vi "内泄露.vi"(0 "内泄漏曲线":refnum<vi>, 1 "内泄漏":cluster{"下限":dbl, "上限":dbl}, 3 "错误输入":errorcluster) -> (8 "OK？":bool, 10 "错误输出":errorcluster)   [LabVIEW 2018]
uses:
  Global_Variable/Global.vi
  Global_Variable/A180648.vi
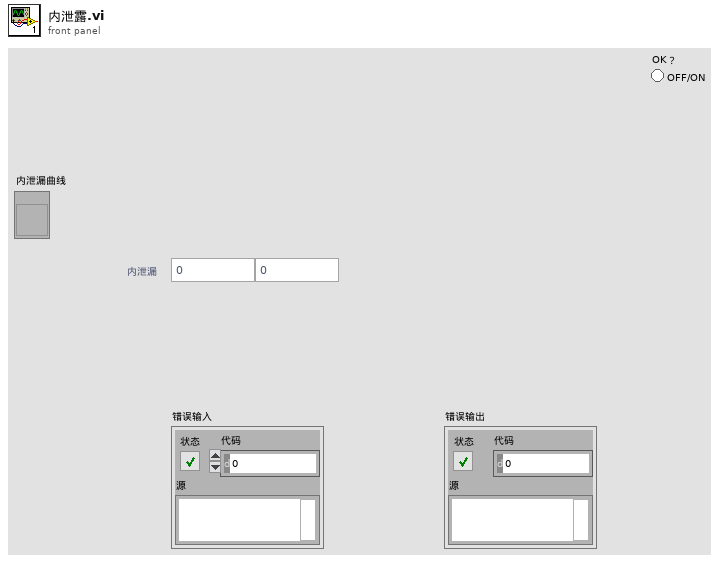
[diagram p1: front panel]
types:
  T1 = enum32{"空载", "功能", "力特性", "传感器特性", "电流特性", "振动NVH", "逆向空载", "完成"}
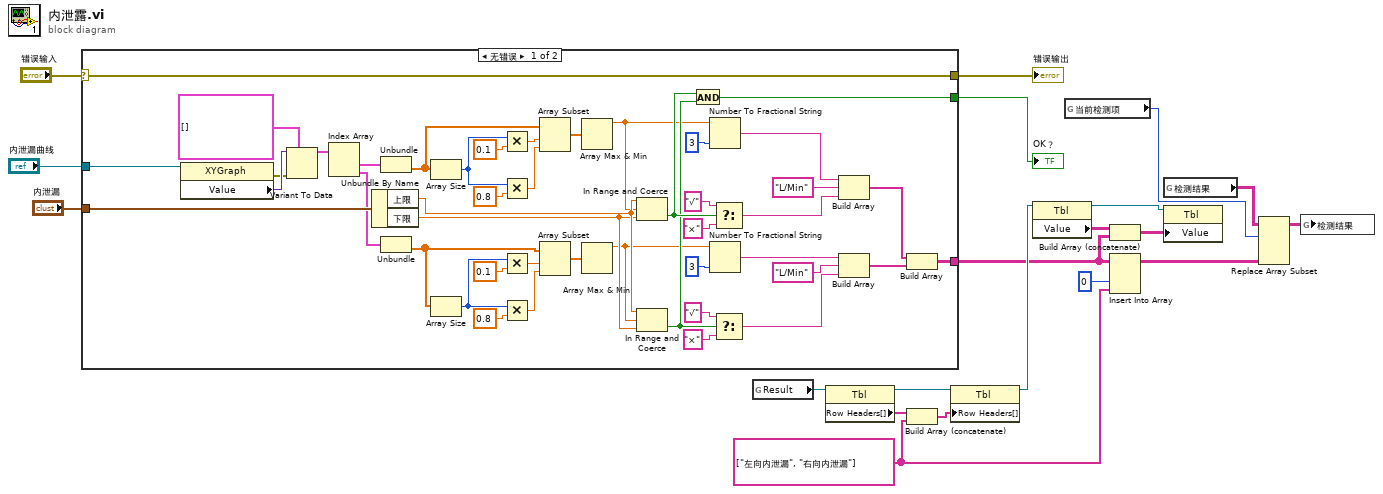
[diagram p0: block diagram]
diagram:
  w3 = string[] ["左向内泄漏", "右向内泄漏"] ("列首字符串[]")
  n1 = case shown="无错误" "错误输入" {
    selector: "错误输入" -> [w44 w66]
    tunnel: [w44 w66] -> w19
    tunnel: [w46 _] -> w18
    tunnel: "内泄漏" -> [w58 _]
    tunnel: [w59 _] -> w4
    tunnel: "内泄漏曲线" -> [w39 _]
    frame No Error {
      n2 = property class="XYGraph"(reference=w39) -> (error out=w42:errorcluster, "Value"=w43:variant)  [unwired: 1 in, 1 out]
      n3 = Variant To Data(error in=w42, type=cluster{dbl[], dbl[]}[] [], Variant=w43) -> (data=w41:cluster{dbl[], dbl[]}[])  [unwired: 1 out]
      n4 = Index Array(array=w41) -> (element #1=w38:cluster{dbl[], dbl[]}, element #2=w37:cluster{dbl[], dbl[]})  [unwired: 2 in]
      n5 = Unbundle By Name(w58) -> ("上限"=w51:dbl, "下限"=w50:dbl)
      n6 = Unbundle(w38) -> (w35:dbl[])  [unwired: 1 out]
      n7 = Unbundle(w37) -> (w23:dbl[])  [unwired: 1 out]
      n8 = Array Size(array=w35) -> (size(s)=w32:i32)
      n9 = Array Size(array=w23) -> (size(s)=w24:i32)
      n10 = Multiply(x=w32, y=0.1) -> (x*y=w30:dbl)
      n11 = Multiply(x=w32, y=0.8) -> (x*y=w29:dbl)
      n12 = Multiply(x=w24, y=0.1) -> (x*y=w26:dbl)
      n13 = Multiply(x=w24, y=0.8) -> (x*y=w27:dbl)
      n14 = Array Subset(array=w35, index=w30, length=w29) -> (w28:dbl[])
      n15 = Array Subset(array=w23, index=w26, length=w27) -> (w21:dbl[])
      n16 = Array Max & Min(array=w28) -> (max value=w34:dbl)  [unwired: 3 out]
      n17 = Array Max & Min(array=w21) -> (max value=w36:dbl)  [unwired: 3 out]
      n18 = In Range and Coerce(upper limit=w51, x=w34, lower limit=w50) -> (In Range?=w48:bool)  [unwired: 1 out]
      n19 = In Range and Coerce(upper limit=w51, x=w36, lower limit=w50) -> (In Range?=w47:bool)  [unwired: 1 out]
      n20 = And(x=w48, y=w47) -> (x .and. y?=w46:bool)
      n21 = Number To Fractional String(number=w34, precision (6)=i16 3 ("精度(6)")) -> (F-format string=w45:string)  [unwired: 2 in]
      n22 = Number To Fractional String(number=w36, precision (6)=i16 3 ("精度(6)")) -> (F-format string=w53:string)  [unwired: 2 in]
      n23 = Select(t="√" ("元素"), s=w48, f="×" ("元素")) -> (s? t:f=w61:string)
      n24 = Select(t="√" ("元素"), s=w47, f="×" ("元素")) -> (s? t:f=w57:string)
      n25 = Build Array(w45, "L/Min" ("元素"), w61) -> (w60:string[])
      n26 = Build Array(w53, "L/Min" ("元素"), w57) -> (w49:string[])
      n27 = Build Array(w60, w49) -> (w59:string[][])
    }
    frame Error {
    }
  }
  "错误输出" <- w19
  "OK？" <- w18
  n28 = global read "Global.vi" "Result"() -> (w14:refnum<vi>)
  n29 = property class="Tbl"(reference=w14) -> (reference out=w13:refnum<vi>, "Row Headers[]"=w11:string[])  [unwired: 1 in, 1 out]
  n30 = Build Array (concatenate)(w11, w3) -> (w10:string[])
  n31 = property class="Tbl"(reference=w13, "Row Headers[]"=w10) -> (reference out=w12:refnum<vi>)  [unwired: 1 in, 1 out]
  n32 = property class="Tbl"(reference=w12) -> (reference out=w17:refnum<vi>, "Value"=w16:string[][])  [unwired: 1 in, 1 out]
  n33 = global read "A180648.vi" "当前检测项"() -> (w7:T1)
  n34 = Build Array (concatenate)(w16, w4) -> (w15:string[][])
  n35 = Insert Into Array(array=w4, index (col)=0 ("禁用的索引 (列)"), new element=w3) -> (w1:string[][])  [unwired: 1 in]
  n36 = global read "A180648.vi" "检测结果"() -> (w8:string[][][])
  n37 = property class="Tbl"(reference=w17, "Value"=w15) -> ()  [unwired: 1 in, 2 out]
  n38 = Replace Array Subset(array=w8, new element=w1, index (dim 0)=w7) -> (w6:string[][][])  [unwired: 2 in]
  n39 = global write "A180648.vi" "检测结果"(w6) -> ()
